vi "CvrtCell2Data.vi"(8 "error in (no error)":errorcluster, 9 "ge_HdrNames":T1, 10 "Item Name":string, 11 "Strain in":refnum<class "Strain.lvclass">) -> (0 "error out":errorcluster, 3 "Strain out":refnum<class "Strain.lvclass">)   [LabVIEW 2012, in "Measurement Channels.lvlib" / "Strain.lvclass"]
uses:
  Strain.lvclass
  Common/Controls/HeaderNames.ctl
  Class Channel/Channel.lvclass
  SubVIs Table/Custom Ctls Table/ge_ColType.ctl
  Strain.lvclass/Strain.ctl
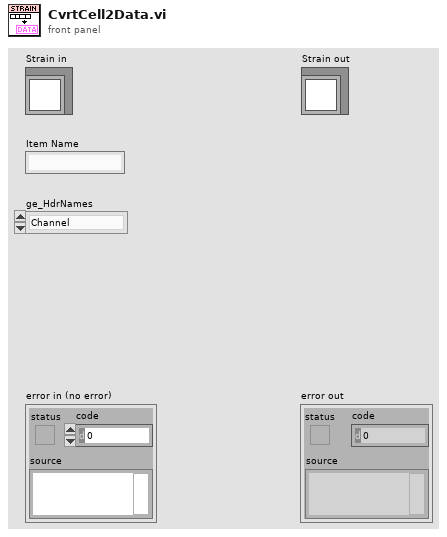
[diagram p1: front panel]
types:
  T1 = typedef "HeaderNames.ctl" = enum16{"Channel", "Device", "Spacer", "Description", "MB", "Range", "Terminal", "Coupling", "Thresh (V)", "Pulse/Rev", "Slope", "Min EU", "Min RPM", "mV/EU", "Iex", "Temp Units", "Type", "CJC Src", "CJC Val", "Ro", "Wire Cfg", "Strain Mode", "Vex", "Bridge Type", "GF", "Gauge Res", "Poisson", "Lead Res", "Init Strain", "GAF", "Scale", "Offset", "Unit (EU)", "dB?", "dB Ref", "Cal Mag", "Cal Units", "Max Temp", "Min Temp", "Max Strain", "Min Strain"}
  T2 = typedef "ge_ColType.ctl" = enum16{"Volts", "Amps", "Ohms", "TermCfg", "WireCfg", "Coup", "Slope", "Iex", "CalUnits", "ThrmUnits", "ThrmType", "CJCSrc", "BrdgType", "Strn Mode", "RTDType"}
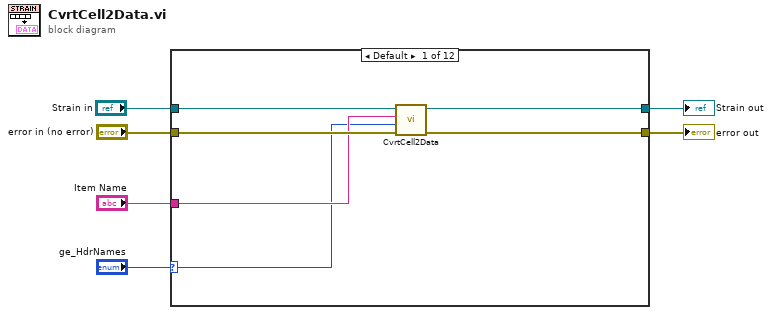
[diagram p0: block diagram]
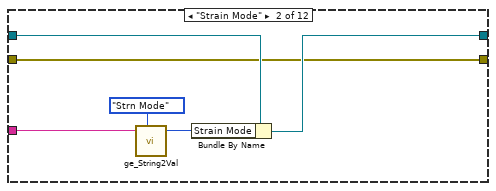
[diagram p2: hidden frame]
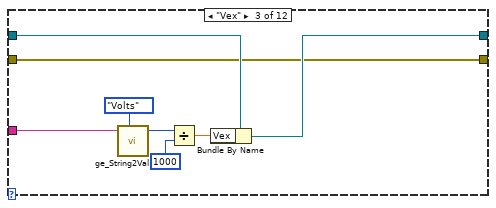
[diagram p3: hidden frame]
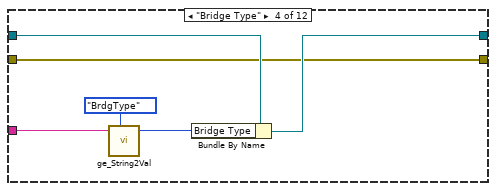
[diagram p4: hidden frame]
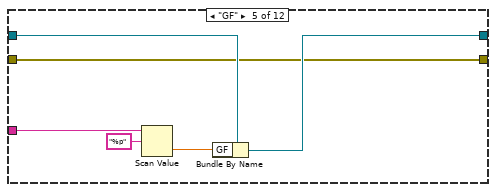
[diagram p5: hidden frame]
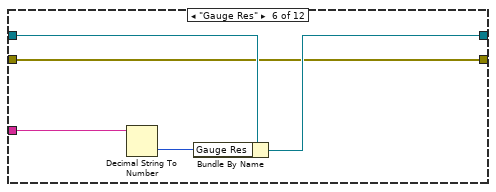
[diagram p6: hidden frame]
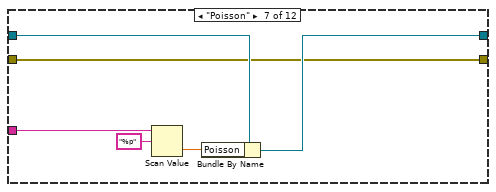
[diagram p7: hidden frame]
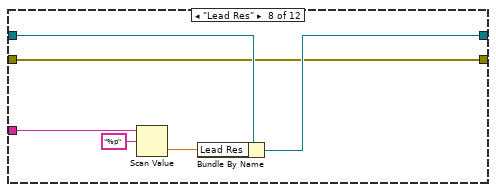
[diagram p8: hidden frame]
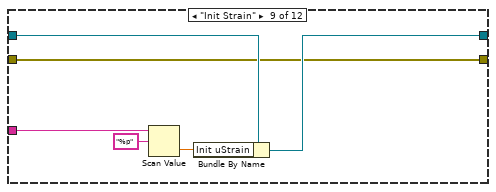
[diagram p9: hidden frame]
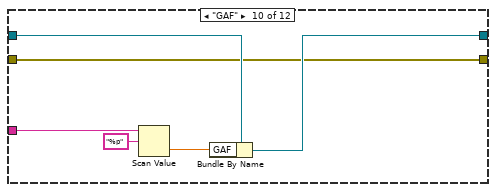
[diagram p10: hidden frame]
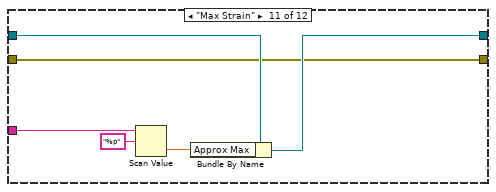
[diagram p11: hidden frame]
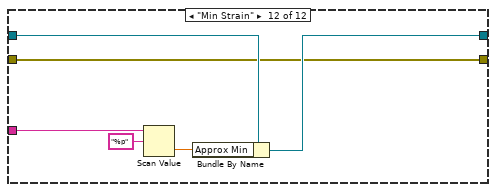
[diagram p12: hidden frame]
diagram:
  n1 = case shown="Default" "ge_HdrNames" {
    selector: "ge_HdrNames" -> [w7 _ _ _ _ _ _ _ _ _ _ _]
    tunnel: [w12 w16 w24 w30 w36 w41 w47 w53 w59 w65 w71 w77] -> w6
    tunnel: [w11 w17 w25 w31 w37 w42 w48 w54 w60 w66 w72 w78] -> w5
    tunnel: "error in (no error)" -> [w10 w16 w24 w30 w36 w41 w47 w53 w59 w65 w71 w77]
    tunnel: "Item Name" -> [w9 w14 w22 w28 w34 w39 w45 w51 w57 w63 w69 w75]
    tunnel: "Strain in" -> [w8 w18 w26 w32 w38 w43 w49 w55 w61 w67 w73 w79]
    frame Default {
      n2 = call-parent "CvrtCell2Data.vi"("error in (no error)"=w10, "Header Names"=w7, "Item Name"=w9, "Channel in"=w8) -> ("error out"=w12:errorcluster, "Channel out"=w11:refnum<class "Strain.lvclass">)  [unwired: 6 in]
    }
    frame "Strain Mode" {
      n3 = call "ge_String2Val.vi"("String"=w14, "ColType"=ge_ColType."Strn Mode") -> ("Value"=w13:u16)  [unwired: 4 in, 1 out]
      n4 = Bundle By Name(cluster=w18, "Strain Mode"=w13) -> (w17:refnum<class "Strain.lvclass">)
    }
    frame "Vex" {
      n5 = call "ge_String2Val.vi"("String"=w22, "ColType"=ge_ColType."Volts") -> ("Value"=w21:u16)  [unwired: 4 in, 1 out]
      n6 = Divide(x=w21, y=1000) -> (x/y=w19:dbl)
      n7 = Bundle By Name(cluster=w26, "Vex"=w19) -> (w25:refnum<class "Strain.lvclass">)
    }
    frame "Bridge Type" {
      n8 = call "ge_String2Val.vi"("String"=w28, "ColType"=ge_ColType."BrdgType") -> ("Value"=w27:u16)  [unwired: 4 in, 1 out]
      n9 = Bundle By Name(cluster=w32, "Bridge Type"=w27) -> (w31:refnum<class "Strain.lvclass">)
    }
    frame "GF" {
      n10 = Scan Value(string=w34, format string="%p") -> (value=w33:dbl)  [unwired: 1 in, 1 out]
      n11 = Bundle By Name(cluster=w38, "GF"=w33) -> (w37:refnum<class "Strain.lvclass">)
    }
    frame "Gauge Res" {
      n12 = Decimal String To Number(string=w39) -> (number=w40:i32)  [unwired: 2 in, 1 out]
      n13 = Bundle By Name(cluster=w43, "Gauge Res"=w40) -> (w42:refnum<class "Strain.lvclass">)
    }
    frame "Poisson" {
      n14 = Scan Value(string=w45, format string="%p") -> (value=w44:dbl)  [unwired: 1 in, 1 out]
      n15 = Bundle By Name(cluster=w49, "Poisson"=w44) -> (w48:refnum<class "Strain.lvclass">)
    }
    frame "Lead Res" {
      n16 = Scan Value(string=w51, format string="%p") -> (value=w50:dbl)  [unwired: 1 in, 1 out]
      n17 = Bundle By Name(cluster=w55, "Lead Res"=w50) -> (w54:refnum<class "Strain.lvclass">)
    }
    frame "Init Strain" {
      n18 = Scan Value(string=w57, format string="%p") -> (value=w56:dbl)  [unwired: 1 in, 1 out]
      n19 = Bundle By Name(cluster=w61, "Init uStrain"=w56) -> (w60:refnum<class "Strain.lvclass">)
    }
    frame "GAF" {
      n20 = Scan Value(string=w63, format string="%p") -> (value=w62:dbl)  [unwired: 1 in, 1 out]
      n21 = Bundle By Name(cluster=w67, "GAF"=w62) -> (w66:refnum<class "Strain.lvclass">)
    }
    frame "Max Strain" {
      n22 = Scan Value(string=w69, format string="%p") -> (value=w68:dbl)  [unwired: 1 in, 1 out]
      n23 = Bundle By Name(cluster=w73, "Approx Max"=w68) -> (w72:refnum<class "Strain.lvclass">)
    }
    frame "Min Strain" {
      n24 = Scan Value(string=w75, format string="%p") -> (value=w74:dbl)  [unwired: 1 in, 1 out]
      n25 = Bundle By Name(cluster=w79, "Approx Min"=w74) -> (w78:refnum<class "Strain.lvclass">)
    }
  }
  "error out" <- w6
  "Strain out" <- w5
